vi "Main_FSM.vi"() -> ()   [LabVIEW 2018]
uses:
  F:/Program Files (x86)/National Instruments/LabVIEW 2018/examples/Instrument IO/Serial/support/Serial - Settings.ctl
  Control/serial.ctl
panel:
  out "state":u16
  in  "CMD 쓰기":bool
  in  "시작":bool
  out "Response":string
  in  "Command":string="*IDN?"
  in  "Serial Settings":T1={"baud rate"=9600, "data bits"=8, "parity"=enum."None", "stop bits"=10, "flow control"=0} {"flow control" items=["None"=0, "XON/XOFF"=1, "RTS/CTS"=2, "DTR/DSR"=4]; "stop bits" items=["1.0"=10, "1.5"=15, "2.0"=20]; "data bits" min=5 max=8 step=1; "baud rate" items=["75"=75, "110"=110, "134"=134, "150"=150, "300"=300, "600"=600, "1200"=1200, "1800"=1800, "2400"=2400, "4800"=4800, "7200"=7200, "9600"=9600, "14400"=14400, "19200"=19200, "28800"=28800, "38400"=38400, "56000"=56000, "57600"=57600, "115200"=115200, "128000"=128000, "230400"=230400]}
  in  "VISA resource name":refnum<visa-resource-name>="COM1"
  in  "정지":bool
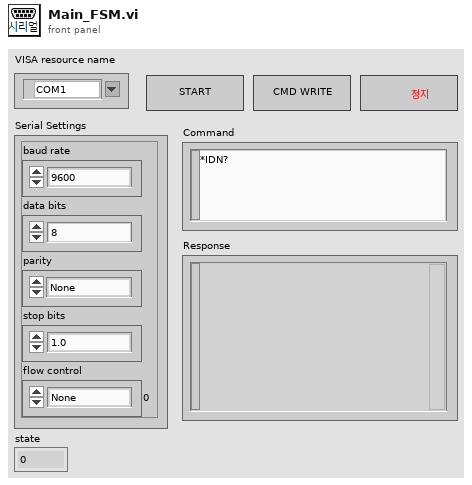
[diagram p1: front panel]
types:
  T1 = typedef "Serial - Settings.ctl" = cluster{"baud rate":u32, "data bits":u16, "parity":enum16{"None", "Odd", "Even", "Mark", "Space"}, "stop bits":u16, "flow control":u16}
  T2 = typedef "상태.ctl" = enum16{"대기", "설정", "초기화", "읽기", "쓰기", "정지"}
  T3 = typedef "serial.ctl" = enum16{"설정", "읽기", "쓰기", "종료"}
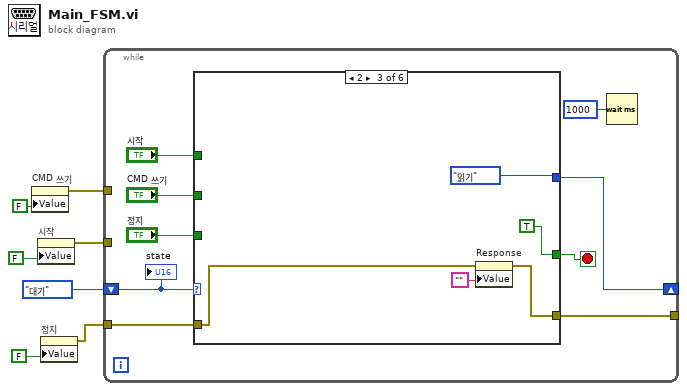
[diagram p0: block diagram]
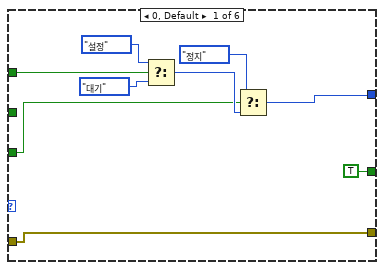
[diagram p2: hidden frame]
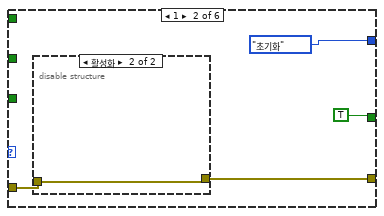
[diagram p3: hidden frame]
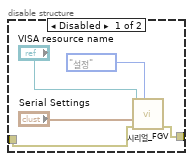
[diagram p4: hidden frame]
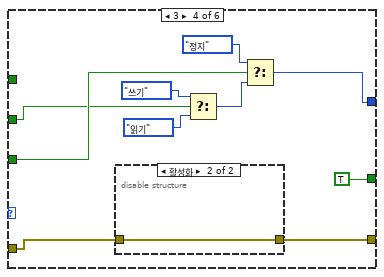
[diagram p5: hidden frame]
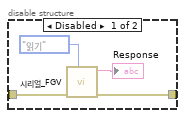
[diagram p6: hidden frame]
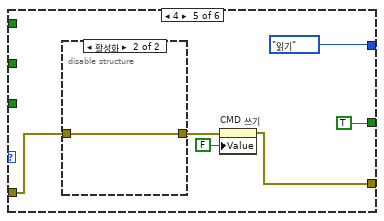
[diagram p7: hidden frame]
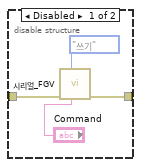
[diagram p8: hidden frame]
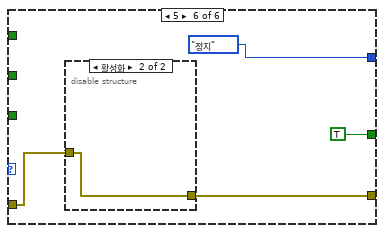
[diagram p9: hidden frame]
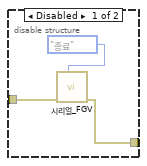
[diagram p10: hidden frame]
diagram:
  n1 = property on="CMD 쓰기" class="Bool (엄격한)"("Value"=FALSE ("CMD 쓰기")) -> (error out=w3:errorcluster)  [unwired: 2 in, 1 out]
  n2 = property on="시작" class="Bool (엄격한)"("Value"=FALSE ("시작")) -> (error out=w1:errorcluster)  [unwired: 2 in, 1 out]
  n3 = property on="정지" class="Bool (엄격한)"("Value"=FALSE ("정지")) -> (error out=w2:errorcluster)  [unwired: 2 in, 1 out]
  n4 = while {
    shift-right: [w12] -> _
    shift-left: 상태."대기" ("상태") -> [w16]
    tunnel: w2 -> [w11]
    tunnel: [w10] -> _
    tunnel: w3 -> [_]
    tunnel: w1 -> [_]
    stop <- w9 stop-if-true
    n5 = case shown="2" w16 {
      tunnel: "시작" -> [w25 _ _ _ _ _]
      tunnel: "CMD 쓰기" -> [_ _ _ w45 _ _]
      tunnel: "정지" -> [w21 _ _ w48 _ _]
      tunnel: [w19 상태."초기화" ("상태") 상태."읽기" ("상태") w42 serial."읽기" ("state") 상태."정지" ("상태")] -> w12
      tunnel: w11 -> [w18 w29 w36 w50 w61 w68]
      tunnel: [w18 w28 w40 w49 w58 w67] -> w10
      tunnel: [TRUE TRUE TRUE TRUE TRUE TRUE] -> w9
      frame 0, Default {
        n6 = Select(t=상태."설정" ("상태"), s=w25, f=상태."대기" ("상태")) -> (s? t:f=w22:T2)
        n7 = Select(t=상태."정지" ("상태"), s=w21, f=w22) -> (s? t:f=w19:T2)
      }
      frame 1 {
        n8 = disable-structure shown="활성화" {
          disable-tunnel: w29 -> [w31 w35]
          disable-tunnel: [w30 w35] -> w28
          frame Disabled {
            n9 = call "시리얼_FGV.vi"("state"=serial."설정", "Error In"=w31, "Serial Settings"="Serial Settings", "VISA resource name"="VISA resource name") -> ("Error Out"=w30:errorcluster)  [unwired: 6 in, 1 out]
          }
          frame Enabled {
          }
        }
      }
      frame 2 {
        n10 = property on="Response" class="Str"(error in=w36, "Value"="") -> (error out=w40:errorcluster)  [unwired: 1 in, 1 out]
      }
      frame 3 {
        n11 = disable-structure shown="활성화" {
          disable-tunnel: w50 -> [w52 w55]
          disable-tunnel: [w51 w55] -> w49
          frame Disabled {
            n12 = call "시리얼_FGV.vi"("state"=serial."읽기", "Error In"=w52) -> ("Error Out"=w51:errorcluster, "Response"=→"Response":string)  [unwired: 8 in]
          }
          frame Enabled {
          }
        }
        n13 = Select(t=상태."쓰기" ("상태"), s=w45, f=상태."읽기" ("상태")) -> (s? t:f=w46:T2)
        n14 = Select(t=상태."정지" ("상태"), s=w48, f=w46) -> (s? t:f=w42:T2)
      }
      frame 4 {
        n15 = disable-structure shown="활성화" {
          disable-tunnel: w61 -> [w63 w66]
          disable-tunnel: [w62 w66] -> w60
          frame Disabled {
            n16 = call "시리얼_FGV.vi"("Command"="Command", "state"=serial."쓰기", "Error In"=w63) -> ("Error Out"=w62:errorcluster)  [unwired: 7 in, 1 out]
          }
          frame Enabled {
          }
        }
        n17 = property on="CMD 쓰기" class="Bool (엄격한)"(error in=w60, "Value"=FALSE ("CMD 쓰기")) -> (error out=w58:errorcluster)  [unwired: 1 in, 1 out]
      }
      frame 5 {
        n18 = disable-structure shown="활성화" {
          disable-tunnel: w68 -> [w72 w74]
          disable-tunnel: [w71 w74] -> w67
          frame Disabled {
            n19 = call "시리얼_FGV.vi"("state"=serial."종료", "Error In"=w72) -> ("Error Out"=w71:errorcluster)  [unwired: 8 in, 1 out]
          }
          frame Enabled {
          }
        }
      }
    }
    n20 = Wait (ms)(milliseconds to wait=u32 1000 ("대기 시간 (ms)")) -> ()  [unwired: 1 out]
    "state" <- w16
  }
